vi "Initialize ANC350v4, and read Axis-1 info..vi"() -> ()   [LabVIEW 2024, in "SampleRotator.lvlib"]
uses:
  SampleRotator.lvlib
  ctl/Rotator controller info.ctl
  ctl/Axis status.ctl
panel:
  out "search":u32
  out "dev info":u32
  out "x-y":u32
  out "Axis status":T1
  in  "Path to *.DLL":path
  out "ANC350v4_Handle_Out":i32
  out "output cluster":T2 {"DeviceType" items=["ANC350res", "ANC350num", "ANC350fps", "No device / invalid"]; "ID" format="%x"}
  out "ANC350v4 found":u32
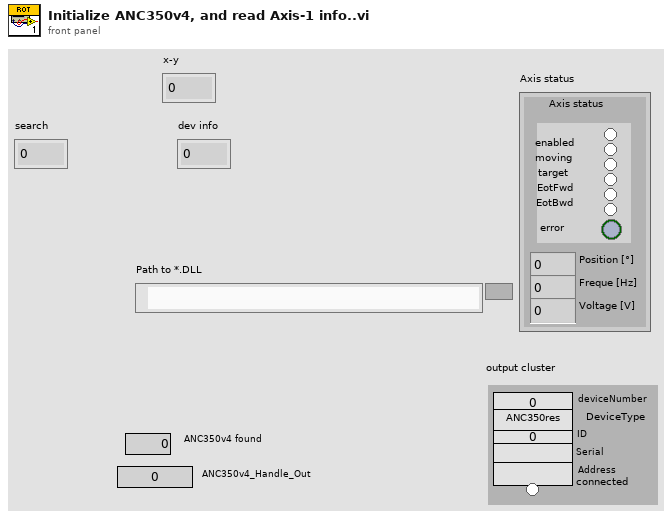
[diagram p1: front panel]
types:
  T1 = typedef "SampleRotator.lvlib/Axis status.ctl" = cluster{"Axis status":cluster{"connected":bool, "enabled":bool, "moving":bool, "target":bool, "EotFwd":bool, "EotBwd":bool, "error":bool}, "Position [°]":dbl, "Freque [Hz]":dbl, "Voltage [V]":dbl}
  T2 = typedef "SampleRotator.lvlib/Rotator controller info.ctl" = cluster{"deviceNumber":i32, "DeviceType":i32, "ID":u32, "Serial":string, "Address":string, "connected":bool}
  T3 = cluster{"deviceNumber":i32, "DeviceType":i32, "ID":u32, "Serial":string, "Address":string, "connected":bool}
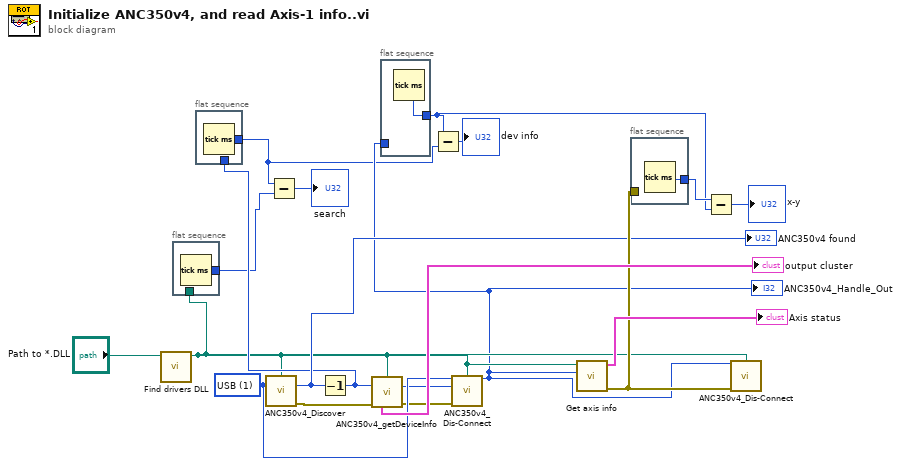
[diagram p0: block diagram]
diagram:
  w17 = u32 1 items=["None", "USB", "TCP", "All"] ("Interface types")
  n1 = call "Find drivers DLL.vi"("Path to DLL"="Path to *.DLL") -> ("path out"=w4:path)  [unwired: 8 in, 2 out]
  n2 = flat-sequence {
    tunnel: [w20] -> w6
    tunnel: w4 -> [_]
    frame #0 {
      n3 = Tick Count (ms)() -> (millisecond timer value=w20:u32)
    }
  }
  n4 = flat-sequence {
    tunnel: [w21] -> w2
    tunnel: w7 -> [_]
    frame #0 {
      n5 = Tick Count (ms)() -> (millisecond timer value=w21:u32)
    }
  }
  n6 = call <instrlib>:"ANC350v4_Discover.vi"("Path to *.DLL"=w4, "Interface types"=w17) -> ("ANC350v4 found"=w8:u32, "error ANC350v4_discover"=w19:errorcluster)  [unwired: 12 in]
  "ANC350v4 found" <- w8
  n7 = Subtract(x=w2, y=w6) -> (x-y=→"search":u32)
  n8 = Decrement(x=w8) -> (x-1=w7:u32)
  n9 = call <instrlib>:"ANC350v4_getDeviceInfo.vi"("Path to *.DLL"=w4, "deviceNumber"=w7, "error in"=w19) -> ("deviceNumber"=w5:i32, "output cluster"=→"output cluster":T3, "Error_ANC350v4_getDeviceInfo"=w16:errorcluster)  [unwired: 5 in, 5 out]
  n10 = flat-sequence {
    tunnel: [w23] -> w1
    tunnel: w3 -> [w22]
    tunnel: [w22] -> _
    frame #0 {
      n11 = Tick Count (ms)() -> (millisecond timer value=w23:u32)
    }
  }
  n12 = Subtract(x=w1, y=w2) -> (x-y=→"dev info":u32)
  n13 = call <instrlib>:"ANC350v4_Dis-Connect.vi"("ANC350v4_Handle"=w17, "Path to *.DLL"=w4, "deviceNumber"=w5, "error in"=w16) -> ("ANC350v4_Handle_Out"=w3:i32)  [unwired: 10 in, 1 out]
  "ANC350v4_Handle_Out" <- w3
  n14 = call "Get axis info.vi"("deviceHandle"=w3, "path in"=w4) -> ("error out"=w13:errorcluster, "Axis status"=→"Axis status":T1)  [unwired: 6 in, 2 out]
  n15 = flat-sequence {
    tunnel: [w24] -> w12
    tunnel: w13 -> [_]
    frame #0 {
      n16 = Tick Count (ms)() -> (millisecond timer value=w24:u32)
    }
  }
  n17 = Subtract(x=w12, y=w1) -> (x-y=→"x-y":u32)
  n18 = call <instrlib>:"ANC350v4_Dis-Connect.vi"("ANC350v4_Handle"=w3, "Path to *.DLL"=w4, "error in"=w13) -> ()  [unwired: 11 in, 2 out]
